vi "PhotonPoseEstimator_Update_All.vi"(9 "Has Results":bool, 10 "PipelineResult":T1, 11 "PhotonPoseEstimator":T11) -> (1 "Pos Found":bool, 2 "PhotonEstimatedRobotPose":T2={"EstimatedPose"={"Translation3d"={"X"=0.0, "Y"=0.0, "Z"=0.0}, "Rotation3d"={"Q_quaternion"={"R"=1.0, "V"=[0.0, 0.0, 0.0]}}}, "TimeStamp_Seconds"=0.0, "targetsUsed"=[], "Strategy"=enum."LOWEST_AMBIGUITY"} {"targetsUsed"."AltCameraToTarget"."TRANSLATION3D"."Z" format="%14.3f"; "targetsUsed"."AltCameraToTarget"."TRANSLATION3D"."Y" format="%14.3f"; "targetsUsed"."AltCameraToTarget"."TRANSLATION3D"."X" format="%14.3f"; "targetsUsed"."BestCameraToTarget"."TRANSLATION3D"."Z" format="%14.3f"; "targetsUsed"."BestCameraToTarget"."TRANSLATION3D"."Y" format="%14.3f"; "targetsUsed"."BestCameraToTarget"."TRANSLATION3D"."X" format="%14.3f"; "EstimatedPose"."Translation3d"."Z" format="%14.3f"; "EstimatedPose"."Translation3d"."Y" format="%14.3f"; "EstimatedPose"."Translation3d"."X" format="%14.3f"}, 3 "out PhotonPoseEstimator":T11)   [LabVIEW 2019, in "PhotonVisionLib.lvlib"]
doc: "Provided data from polling a camera, updates the estimated position of the robot. Returns empty if:\n - New data has not been received since the last call to update.\n - No targets were found from the camera\n - There is no camera set\n\n\nInputs:\n -- PhotonPoseEstimator -- data cluster -- Data guiding how the position determination is done.\n -- PipelineResults -- data cluster -- Data provided from PhotonCamera_GetLatestResults.\n -- HasResults -- boolean - TRUE if targets have been identified in the Pipeline results. This can be provided by PhotonCamera_GetLatestResults.\n -- cameraMatrix -- matrix -- Camera calibration data that can be used in the case of no assigned PhotonCamera.\n -- distCoeffs -- matrix -- Camera calibration data that can be used in the case of no assigned PhotonCamera\n\nOutputs:\n -- PhotonPoseEstimator -- data cluster -- Updated data cluster.\n -- PhotonEstimatedRobotPose -- data cluster -- Estimated robot position, timestamp, and targets used to create the estimte.\n -- PosFound -- boolean -- A position has been determined."
uses:
  PhotonVisionLib.lvlib
  <vilib>/Rock Robotics/WPI/ThirdParty/JAS_Junk/TrajLib/TypeDef/TRANSLATION3D.ctl
  <vilib>/Rock Robotics/WPI/ThirdParty/JAS_Junk/TrajLib/Trajectory_Library.lvlib
  <vilib>/Rock Robotics/WPI/ThirdParty/JAS_Junk/TrajLib/TypeDef/QUATERNION.ctl
  <vilib>/Rock Robotics/WPI/ThirdParty/JAS_Junk/TrajLib/TypeDef/ROTATION3D.ctl
  <vilib>/Rock Robotics/WPI/ThirdParty/JAS_Junk/TrajLib/TypeDef/POSE3D.ctl
  TypeDef/PhotonEstimatedRobotPoseType.ctl
  Enum/PhotonPoseStrategy_ENUM.ctl
  TypeDef/TargetCornerType.ctl
  <vilib>/Rock Robotics/WPI/ThirdParty/JAS_Junk/TrajLib/TypeDef/TRANSFORM3D.ctl
  TypeDef/PhotonTrackedTargetType.ctl
  <vilib>/Rock Robotics/WPI/ThirdParty/JAS_Junk/TrajLib/TypeDef/AprilTag.ctl
  <vilib>/Rock Robotics/WPI/ThirdParty/JAS_Junk/TrajLib/Enum/AprilTagFieldLayoutOrignPosition_ENUM.ctl
  <vilib>/Rock Robotics/WPI/ThirdParty/JAS_Junk/TrajLib/TypeDef/AprilTagFieldLayout.ctl
  TypeDef/PhotonPoseEstimatorType.ctl
  TypeDef/PhotonPipelineResultType.ctl
  TypeDef/PhotonPNPResultType.ctl
  TypeDef/PhotonMultiTargetPNPResultType.ctl
  TypeDef/PhotonTargetModel.ctl
  Ref/PhotonPoseEstimator_REF.ctl
  Ref/PhotonPipelineResult_REF.ctl
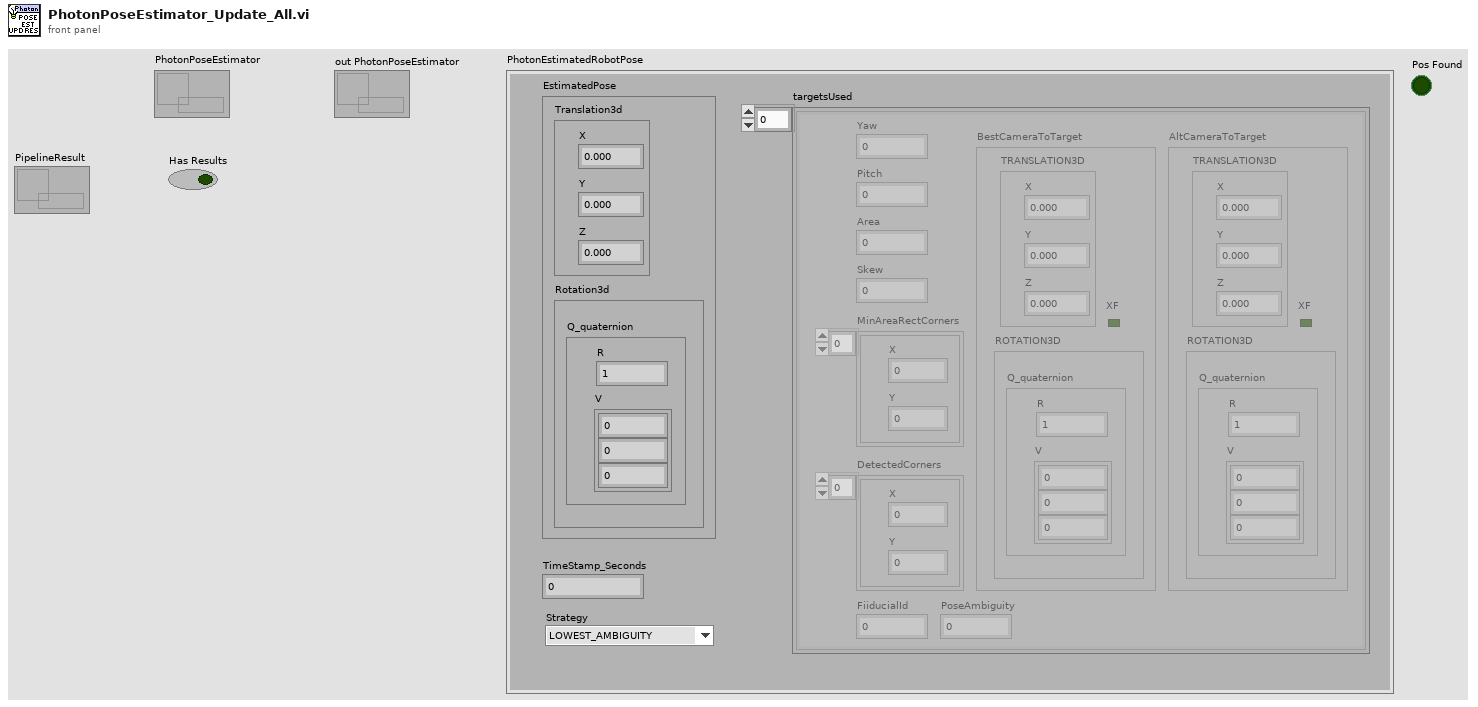
[diagram p1: front panel]
types:
  T1 = typedef "PhotonVisionLib.lvlib/PhotonPipelineResult_REF.ctl" = refnum<data-value>
  T2 = typedef "PhotonVisionLib.lvlib/PhotonEstimatedRobotPoseType.ctl" = cluster{"EstimatedPose":T3, "TimeStamp_Seconds":dbl, "targetsUsed":T7[], "Strategy":T10}
  T3 = typedef "Trajectory_Library.lvlib/POSE3D.ctl" = cluster{"Translation3d":T4, "Rotation3d":T5}
  T4 = typedef "Trajectory_Library.lvlib/TRANSLATION3D.ctl" = cluster{"X":dbl, "Y":dbl, "Z":dbl}
  T5 = typedef "Trajectory_Library.lvlib/ROTATION3D.ctl" = cluster{"Q_quaternion":T6}
  T6 = typedef "Trajectory_Library.lvlib/QUATERNION.ctl" = cluster{"R":dbl, "V":dbl[]}
  T7 = typedef "PhotonVisionLib.lvlib/PhotonTrackedTargetType.ctl" = cluster{"Yaw":dbl, "Pitch":dbl, "Area":dbl, "Skew":dbl, "MinAreaRectCorners":T8[], "BestCameraToTarget":T9, "FiiducialId":i32, "AltCameraToTarget":T9, "PoseAmbiguity":dbl, "DetectedCorners":T8[]}
  T8 = typedef "PhotonVisionLib.lvlib/TargetCornerType.ctl" = cluster{"X":dbl, "Y":dbl}
  T9 = typedef "Trajectory_Library.lvlib/TRANSFORM3D.ctl" = cluster{"TRANSLATION3D":T4, "ROTATION3D":T5, "XF":bool}
  T10 = typedef "PhotonVisionLib.lvlib/PhotonPoseStrategy_ENUM.ctl" = enum16{"LOWEST_AMBIGUITY", "CLOSEST_TO_CAMERA_HEIGHT", "CLOSEST_TO_REFERENCE_POSE", "CLOSEST_TO_LAST_POSE", "AVERAGE_BEST_TARGETS", "MULTI_TAG_PNP_ON_COPROCESSOR", "MULTI_TAG_PNP_ON_RIO"}
  T11 = typedef "PhotonVisionLib.lvlib/PhotonPoseEstimator_REF.ctl" = refnum<data-value>
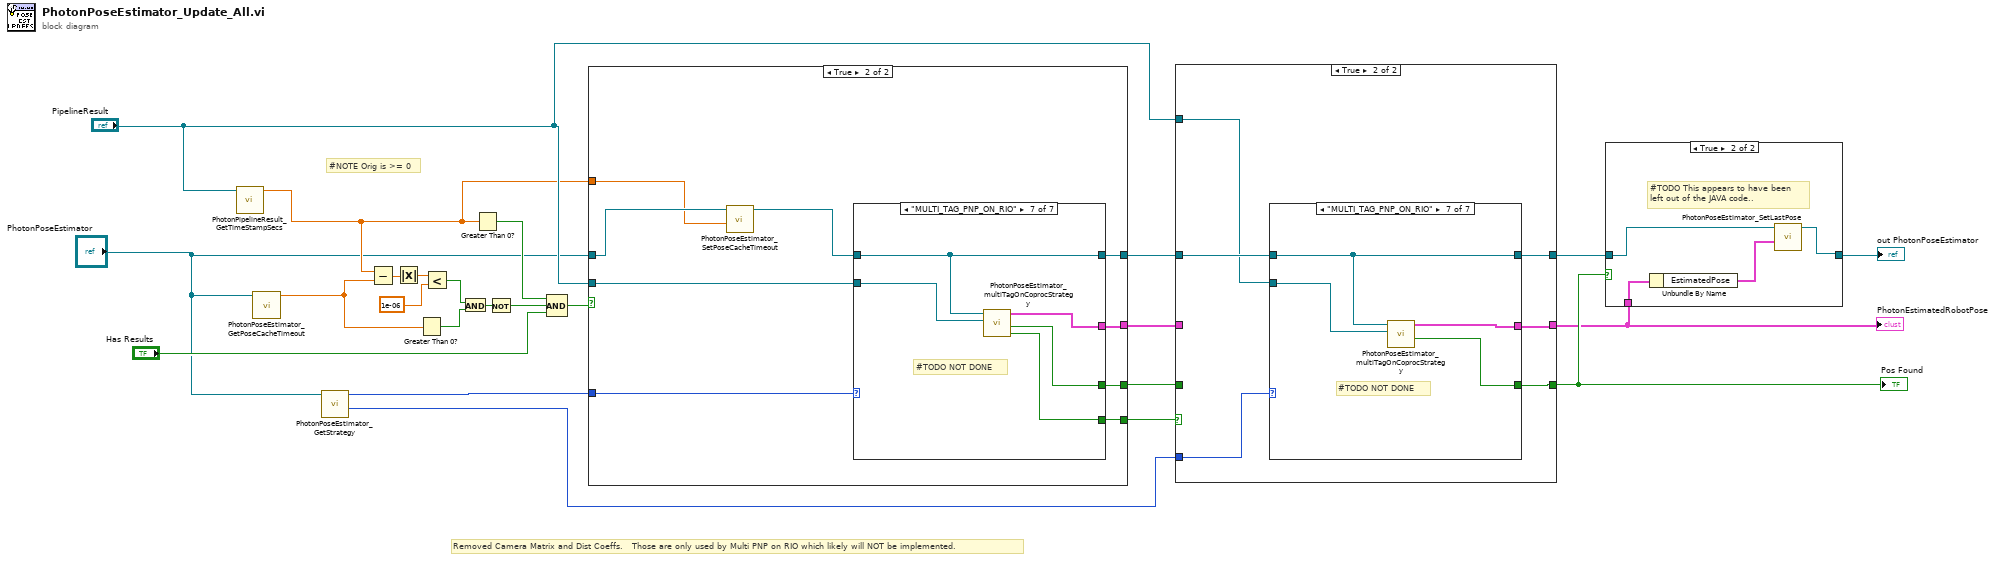
[diagram p0: block diagram]
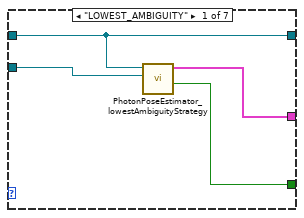
[diagram p3: hidden frame]
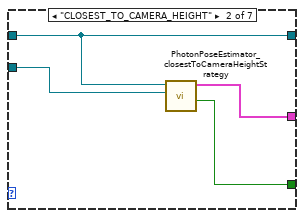
[diagram p4: hidden frame]
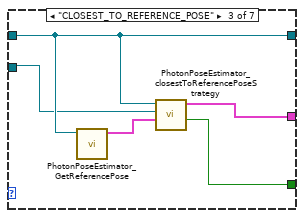
[diagram p5: hidden frame]
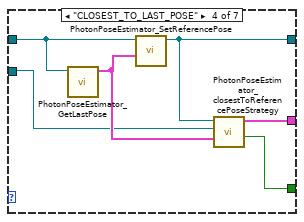
[diagram p6: hidden frame]
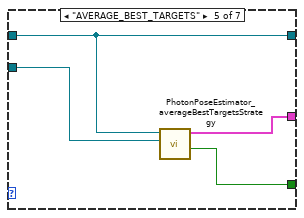
[diagram p7: hidden frame]
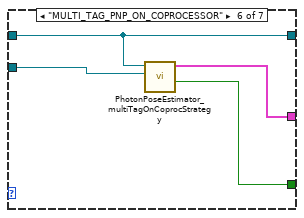
[diagram p8: hidden frame]
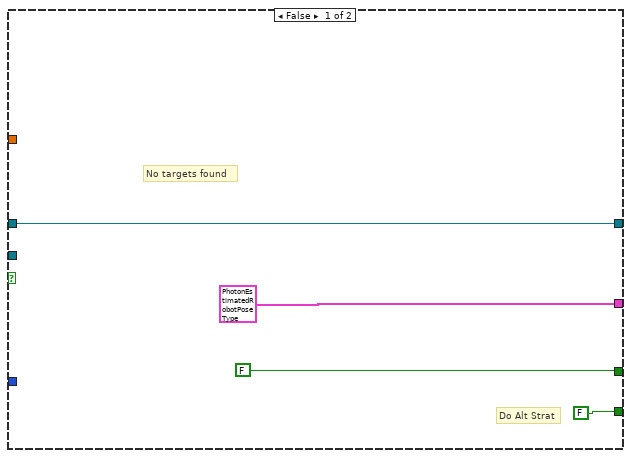
[diagram p9: hidden frame]
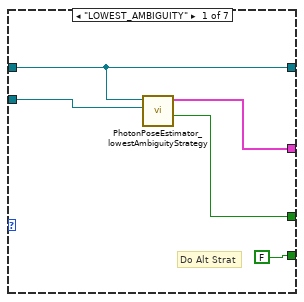
[diagram p10: hidden frame]
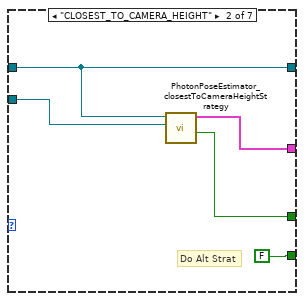
[diagram p11: hidden frame]
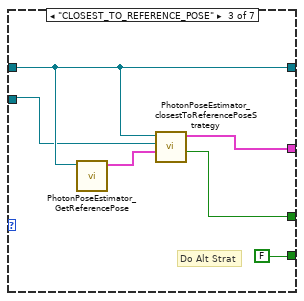
[diagram p12: hidden frame]
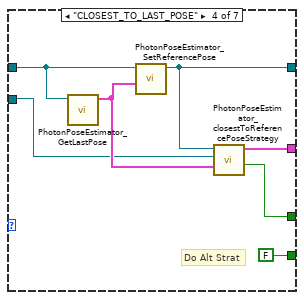
[diagram p13: hidden frame]
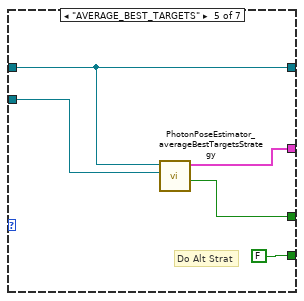
[diagram p14: hidden frame]
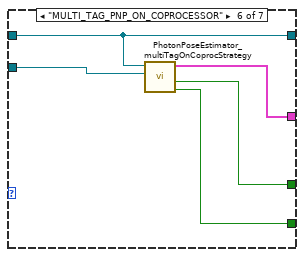
[diagram p15: hidden frame]
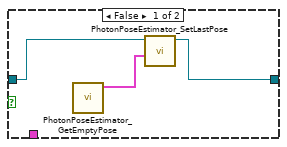
[diagram p16: hidden frame]
diagram:
  # "Removed Camera Matrix and Dist Coeffs.   Those are only used by Multi PNP on RIO which likely will NOT be implemented."
  # "#NOTE Orig is >= 0"
  n1 = call "PhotonPipelineResult_GetTimeStampSecs.vi"("PhotonPipelineResult_REF"="PipelineResult") -> ("TimeStampSec"=w5:dbl)  [unwired: 10 in]
  n2 = call "PhotonPoseEstimator_GetPoseCacheTimeout.vi"("PhotonPoseEstimator"="PhotonPoseEstimator") -> ("PoseCacheTimeoutSec"=w1:dbl)  [unwired: 10 in]
  n3 = call "PhotonPoseEstimator_GetStrategy.vi"("PhotonPoseEstimator"="PhotonPoseEstimator") -> ("MultiTagFallbackStrategy"=w3:T10, "PrimaryStrategy"=w4:T10)  [unwired: 9 in]
  n4 = Subtract(x=w5, y=w1) -> (x-y=w20:dbl)
  n5 = Absolute Value(x=w20) -> (abs(x)=w19:dbl)
  n6 = Greater Than 0?(x=w1) -> (x > 0?=w16:bool)
  n7 = Less?(x=w19, y=1e-06) -> (x < y?=w17:bool)
  n8 = And(x=w17, y=w16) -> (x .and. y?=w15:bool)
  n9 = Greater Than 0?(x=w5) -> (x > 0?=w22:bool)
  n10 = Not(x=w15) -> (.not. x?=w14:bool)
  n11 = Compound Arithmetic op=AND(w22, w14, "Has Results") -> (w23:bool)
  n12 = case shown="True" w23 {
    tunnel: [w28 w35] -> w8
    tunnel: "PhotonPoseEstimator" -> [w28 w31]
    tunnel: [T2 {"EstimatedPose"={"Translation3d"={"X"=0.0, "Y"=0.0, "Z"=0.0}, "Rotation3d"={"Q_quaternion"={"R"=1.0, "V"=[0.0, 0.0, 0.0]}}}, "TimeStamp_Seconds"=0.0, "targetsUsed"=[], "Strategy"=enum."LOWEST_AMBIGUITY"} ("PhotonEstimatedRobotPose") w33] -> w10
    tunnel: [FALSE w34] -> w12
    tunnel: w4 -> [_ w37]
    tunnel: "PipelineResult" -> [_ w36]
    tunnel: w5 -> [_ w29]
    tunnel: [FALSE ("Do Alt Strategy") w32] -> w13
    frame False {
      # "Do Alt Strat"
      # "No targets found"
    }
    frame True {
      n13 = call "PhotonPoseEstimator_SetPoseCacheTimeout.vi"("PoseCacheTimeoutSec"=w29, "PhotonPoseEstimator"=w31) -> ("out PhotonPoseEstimator"=w30:T11)  [unwired: 9 in]
      n14 = case shown="\"MULTI_TAG_PNP_ON_RIO\"" w37 {
        tunnel: w36 -> [w39 w44 w49 w56 w62 w69 w74]
        tunnel: w30 -> [w40 w45 w50 w60 w63 w70 w75]
        tunnel: [w40 w45 w50 w55 w63 w70 w75] -> w35
        tunnel: [w42 w46 w51 w57 w64 w67 w72] -> w34
        tunnel: [w41 w47 w52 w58 w65 w68 w73] -> w33
        tunnel: [FALSE ("Do Alt Strategy") FALSE ("Do Alt Strategy") FALSE ("Do Alt Strategy") FALSE ("Do Alt Strategy") FALSE ("Do Alt Strategy") w66 w71] -> w32
        frame "LOWEST_AMBIGUITY" {
          # "Do Alt Strat"
          n15 = call "PhotonPoseEstimator_lowestAmbiguityStrategy.vi"("CameraResult"=w39, "data value reference"=w40) -> ("Pos Found"=w42:bool, "PhotonEstimatedRobotPose"=w41:T2)  [unwired: 8 in]
        }
        frame "CLOSEST_TO_CAMERA_HEIGHT" {
          # "Do Alt Strat"
          n16 = call "PhotonPoseEstimator_closestToCameraHeightStrategy.vi"("CameraResult"=w44, "PhotonPoseEstimator_REF"=w45) -> ("Pos Found"=w46:bool, "PhotonEstimatedRobotPose"=w47:T2)  [unwired: 8 in]
        }
        frame "CLOSEST_TO_REFERENCE_POSE" {
          # "Do Alt Strat"
          n17 = call "PhotonPoseEstimator_GetReferencePose.vi"("PhotonPoseEstimator"=w50) -> ("ReferencePose"=w53:T3)  [unwired: 10 in]
          n18 = call "PhotonPoseEstimator_closestToReferencePoseStrategy.vi"("ReferencePose"=w53, "CameraResult"=w49, "PhotonPoseEstimator_REF"=w50) -> ("Pos Found"=w51:bool, "PhotonEstimatedRobotPose"=w52:T2)  [unwired: 7 in]
        }
        frame "CLOSEST_TO_LAST_POSE" {
          # "Do Alt Strat"
          n19 = call "PhotonPoseEstimator_GetLastPose.vi"("PhotonPoseEstimator"=w60) -> ("LastPose"=w59:T3)  [unwired: 10 in]
          n20 = call "PhotonPoseEstimator_SetReferencePose.vi"("ReferencePose"=w59, "PhotonPoseEstimator"=w60) -> ("out PhotonPoseEstimator"=w55:T11)  [unwired: 9 in]
          n21 = call "PhotonPoseEstimator_closestToReferencePoseStrategy.vi"("ReferencePose"=w59, "CameraResult"=w56, "PhotonPoseEstimator_REF"=w55) -> ("Pos Found"=w57:bool, "PhotonEstimatedRobotPose"=w58:T2)  [unwired: 7 in]
        }
        frame "AVERAGE_BEST_TARGETS" {
          # "Do Alt Strat"
          n22 = call "PhotonPoseEstimator_averageBestTargetsStrategy.vi"("CameraResult"=w62, "PhotonPoseEstimator_REF"=w63) -> ("Pos Found"=w64:bool, "PhotonEstimatedRobotPose"=w65:T2)  [unwired: 8 in]
        }
        frame "MULTI_TAG_PNP_ON_COPROCESSOR" {
          n23 = call "PhotonPoseEstimator_multiTagOnCoprocStrategy.vi"("CameraResult"=w69, "PhotonPoseEstimator_REF"=w70) -> ("Do Alt Strategy"=w66:bool, "Pos Found"=w67:bool, "PhotonEstimatedRobotPose"=w68:T2)  [unwired: 7 in]
        }
        frame "MULTI_TAG_PNP_ON_RIO" {
          # "#TODO NOT DONE"
          n24 = call "PhotonPoseEstimator_multiTagOnCoprocStrategy.vi"("CameraResult"=w74, "PhotonPoseEstimator_REF"=w75) -> ("Do Alt Strategy"=w71:bool, "Pos Found"=w72:bool, "PhotonEstimatedRobotPose"=w73:T2)  [unwired: 7 in]
        }
      }
    }
  }
  n25 = case shown="True" w13 {
    tunnel: [w78 w79] -> w11
    tunnel: w12 -> [w78 _]
    tunnel: w10 -> [w77 _]
    tunnel: [w77 w80] -> w9
    tunnel: w8 -> [w76 w84]
    tunnel: [w76 w81] -> w7
    tunnel: "PipelineResult" -> [_ w83]
    tunnel: w3 -> [_ w82]
    frame False {
    }
    frame True {
      n26 = case shown="\"MULTI_TAG_PNP_ON_RIO\"" w82 {
        tunnel: w83 -> [w85 w89 w93 w99 w104 w110 w112]
        tunnel: w84 -> [w86 w90 w94 w103 w105 w111 w113]
        tunnel: [w86 w90 w94 w98 w105 w111 w113] -> w81
        tunnel: [w88 w91 w95 w100 w106 w108 w114] -> w79
        tunnel: [w87 w92 w96 w101 w107 w109 w115] -> w80
        frame "LOWEST_AMBIGUITY" {
          n27 = call "PhotonPoseEstimator_lowestAmbiguityStrategy.vi"("CameraResult"=w85, "data value reference"=w86) -> ("Pos Found"=w88:bool, "PhotonEstimatedRobotPose"=w87:T2)  [unwired: 8 in]
        }
        frame "CLOSEST_TO_CAMERA_HEIGHT" {
          n28 = call "PhotonPoseEstimator_closestToCameraHeightStrategy.vi"("CameraResult"=w89, "PhotonPoseEstimator_REF"=w90) -> ("Pos Found"=w91:bool, "PhotonEstimatedRobotPose"=w92:T2)  [unwired: 8 in]
        }
        frame "CLOSEST_TO_REFERENCE_POSE" {
          n29 = call "PhotonPoseEstimator_GetReferencePose.vi"("PhotonPoseEstimator"=w94) -> ("ReferencePose"=w97:T3)  [unwired: 10 in]
          n30 = call "PhotonPoseEstimator_closestToReferencePoseStrategy.vi"("ReferencePose"=w97, "CameraResult"=w93, "PhotonPoseEstimator_REF"=w94) -> ("Pos Found"=w95:bool, "PhotonEstimatedRobotPose"=w96:T2)  [unwired: 7 in]
        }
        frame "CLOSEST_TO_LAST_POSE" {
          n31 = call "PhotonPoseEstimator_GetLastPose.vi"("PhotonPoseEstimator"=w103) -> ("LastPose"=w102:T3)  [unwired: 10 in]
          n32 = call "PhotonPoseEstimator_SetReferencePose.vi"("ReferencePose"=w102, "PhotonPoseEstimator"=w103) -> ("out PhotonPoseEstimator"=w98:T11)  [unwired: 9 in]
          n33 = call "PhotonPoseEstimator_closestToReferencePoseStrategy.vi"("ReferencePose"=w102, "CameraResult"=w99, "PhotonPoseEstimator_REF"=w98) -> ("Pos Found"=w100:bool, "PhotonEstimatedRobotPose"=w101:T2)  [unwired: 7 in]
        }
        frame "AVERAGE_BEST_TARGETS" {
          n34 = call "PhotonPoseEstimator_averageBestTargetsStrategy.vi"("CameraResult"=w104, "PhotonPoseEstimator_REF"=w105) -> ("Pos Found"=w106:bool, "PhotonEstimatedRobotPose"=w107:T2)  [unwired: 8 in]
        }
        frame "MULTI_TAG_PNP_ON_COPROCESSOR" {
          n35 = call "PhotonPoseEstimator_multiTagOnCoprocStrategy.vi"("CameraResult"=w110, "PhotonPoseEstimator_REF"=w111) -> ("Pos Found"=w108:bool, "PhotonEstimatedRobotPose"=w109:T2)  [unwired: 7 in, 1 out]
        }
        frame "MULTI_TAG_PNP_ON_RIO" {
          # "#TODO NOT DONE"
          n36 = call "PhotonPoseEstimator_multiTagOnCoprocStrategy.vi"("CameraResult"=w112, "PhotonPoseEstimator_REF"=w113) -> ("Pos Found"=w114:bool, "PhotonEstimatedRobotPose"=w115:T2)  [unwired: 7 in, 1 out]
        }
      }
    }
  }
  "PhotonEstimatedRobotPose" <- w9
  "Pos Found" <- w11
  n37 = case shown="True" w11 {
    tunnel: w7 -> [w117 w122]
    tunnel: [w118 w121] -> w24
    tunnel: w9 -> [_ w120]
    frame False {
      n38 = call "PhotonPoseEstimator_GetEmptyPose.vi"() -> ("EmptyPose"=w116:T3)  [unwired: 11 in]
      n39 = call "PhotonPoseEstimator_SetLastPose.vi"("LastPose"=w116, "PhotonPoseEstimator"=w117) -> ("out PhotonPoseEstimator"=w118:T11)  [unwired: 9 in]
    }
    frame True {
      # "#TODO This appears to have been\nleft out of the JAVA code.."
      n40 = Unbundle By Name(w120) -> ("EstimatedPose"=w119:T3)
      n41 = call "PhotonPoseEstimator_SetLastPose.vi"("LastPose"=w119, "PhotonPoseEstimator"=w122) -> ("out PhotonPoseEstimator"=w121:T11)  [unwired: 9 in]
    }
  }
  "out PhotonPoseEstimator" <- w24
